vi "36-sub-palindrome-base-10-check.vi"(1 "Number":u64) -> (0 "Number is Palindrome in Base 10?":bool)   [LabVIEW 2021]
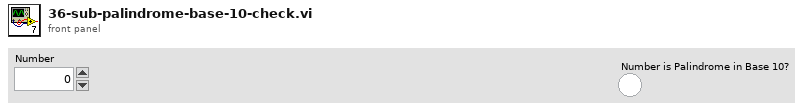
[diagram p1: front panel]
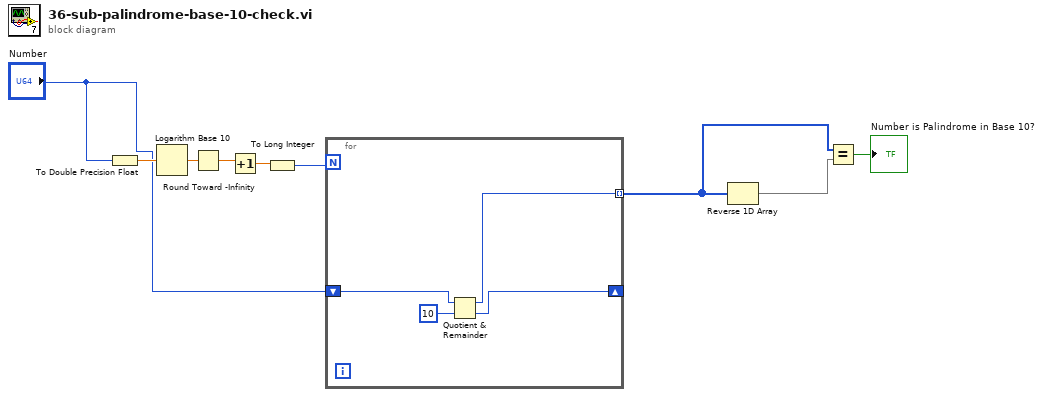
[diagram p0: block diagram]
diagram:
  n1 = To Double Precision Float(number="Number") -> (double precision float=w9:dbl)
  n2 = Logarithm Base 10(1:w9) -> (0:w8:dbl)
  n3 = Round Toward -Infinity(1:w8) -> (0:w7:dbl)
  n4 = Increment(x=w7) -> (x+1=w6:dbl)
  n5 = To Long Integer(number=w6) -> (32bit integer=w3:i32)
  n6 = for {
    N: w3 -> [_]
    shift-right: [w11] -> _
    shift-left: "Number" -> [w13]
    tunnel: [w10] -> w1 mode=indexing
    n7 = Quotient & Remainder(x=w13, y=u64 10) -> (x-y*floor(x/y)=w10:u64, floor(x/y)=w11:u64)
  }
  n8 = Reverse 1D Array(array=w1) -> (reversed array=w5:u64[])
  n9 = Equal?(x=w1, y=w5) -> (x = y?=→"Number is Palindrome in Base 10?":bool)
